vi "Pre Launch Init.vi"(11 "Parent in":refnum<class "Message_Distributor_Class.lvclass">) -> (0 "error out":errorcluster, 3 "Parent out":refnum<class "Message_Distributor_Class.lvclass">)   [LabVIEW 2023, in "Actor_Message_Distributor.lvlib" / "Message_Distributor_Class.lvclass"]
doc: "(<B>Filename</B>: Actor Framework.lvlib:Actor.lvclass:Pre Launch Init.vi)\n\nDefines behavior that occurs after the Launch Nested Actor method is invoked but before the actor's Actor Core method begins running.\n\nBy default, this method does nothing. A descendant class may override it to define behavior."
uses:
  Message_Distributor_Class.lvclass
  Abstraction_Interface_Class/Abstraction_Interface_Class.lvclass
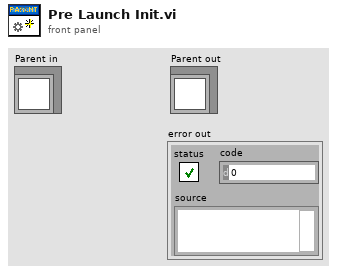
[diagram p1: front panel]
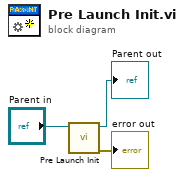
[diagram p0: block diagram]
diagram:
  n1 = call-parent "Pre Launch Init.vi"("Actor in"="Parent in") -> ("error out"=→"error out":errorcluster, "Actor out"=→"Parent out":refnum<class "Message_Distributor_Class.lvclass">)  [unwired: 9 in]
